vi "S3859061_task4.vi"() -> ()   [LabVIEW 2020]
panel:
  out "Waveform Chart":cluster{dbl, dbl}(graph)
  in  "stop":bool
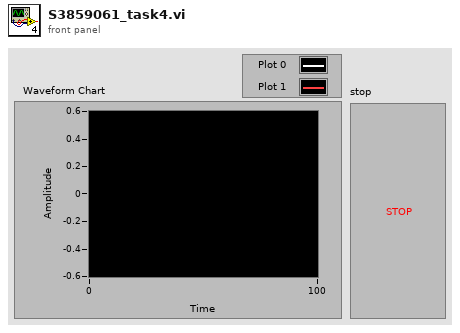
[diagram p1: front panel]
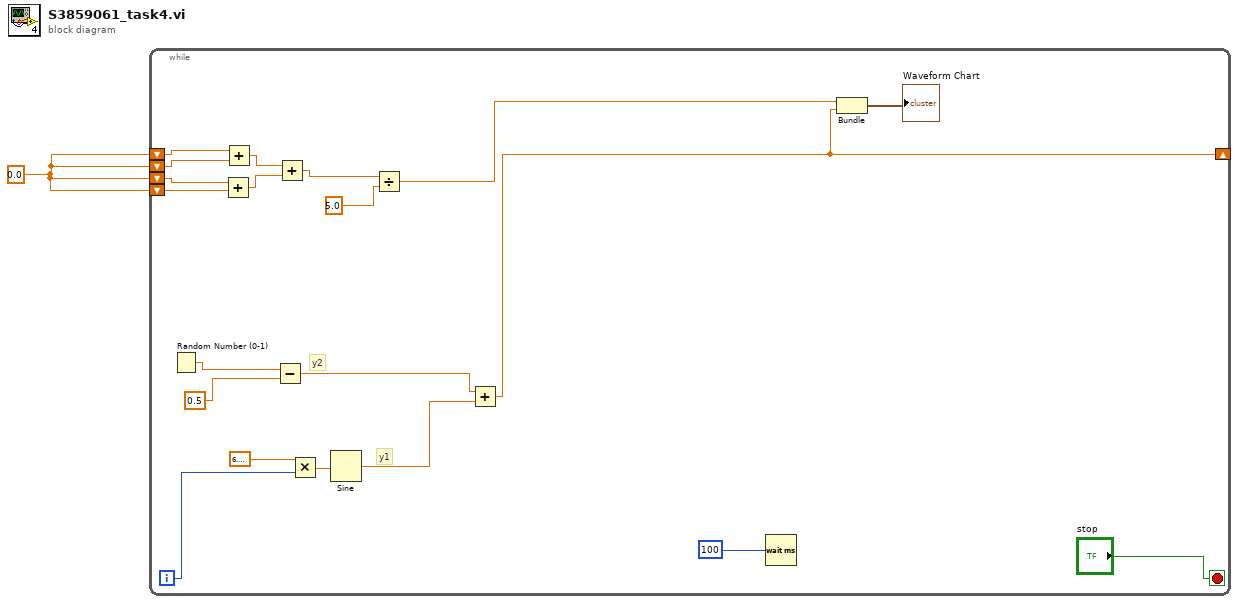
[diagram p0: block diagram]
diagram:
  w1 = 0.0
  n1 = while {
    shift-right: [w3] -> _
    shift-left: w1 -> [w12]
    shift-left: w1 -> [w11]
    shift-left: w1 -> [w10]
    shift-left: w1 -> [w9]
    i -> [w19]
    stop <- "stop" stop-if-true
    # "y1"
    # "y2"
    n2 = Random Number (0-1)() -> (number: 0 to 1=w16:dbl)
    n3 = Add(x=w10, y=w9) -> (x+y=w7:dbl)
    n4 = Add(x=w12, y=w11) -> (x+y=w8:dbl)
    n5 = Subtract(x=w16, y=0.5) -> (x-y=w14:dbl)
    n6 = Add(x=w8, y=w7) -> (x+y=w6:dbl)
    n7 = Multiply(x=6.283185307179586, y=w19) -> (x*y=w17:dbl)
    n8 = Sine(x=w17) -> (sin(x)=w13:dbl)
    n9 = Divide(x=w6, y=5.0) -> (x/y=w4:dbl)
    n10 = Add(x=w14, y=w13) -> (x+y=w3:dbl)
    n11 = Wait (ms)(milliseconds to wait=100) -> ()  [unwired: 1 out]
    n12 = Bundle(w4, w3) -> (→"Waveform Chart":cluster{dbl, dbl})  [unwired: 1 in]
  }
